vi "deleteWrite command description.vi"(8 "error in (no error)":errorcluster, 10 "command description":string, 11 "Help in":refnum<class "Help.lvclass">) -> (0 "error out":errorcluster, 3 "Help out":refnum<class "Help.lvclass">)   [LabVIEW 2019]
uses:
  Help.lvclass
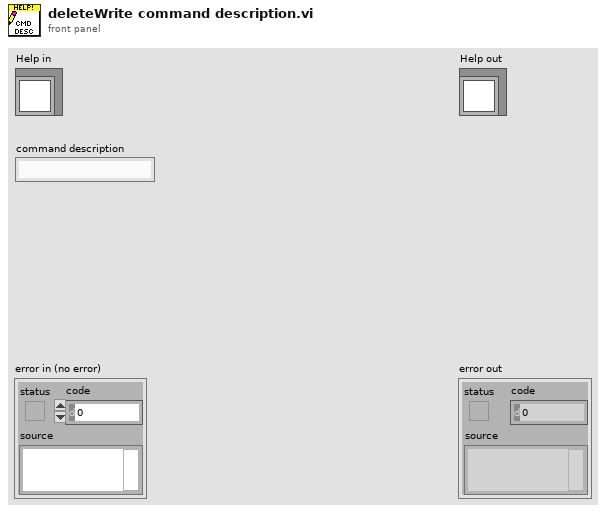
[diagram p1: front panel]
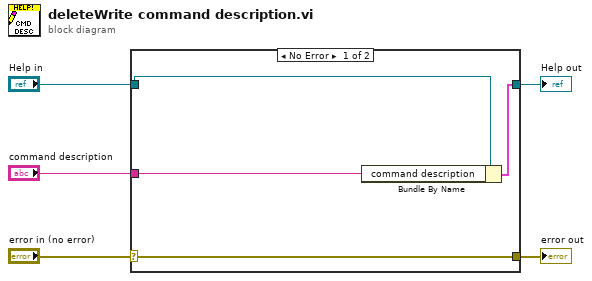
[diagram p0: block diagram]
diagram:
  n1 = case shown="No Error" "error in (no error)" {
    selector: "error in (no error)" -> [w9 w10]
    tunnel: [w9 w10] -> w4
    tunnel: [w7 w11] -> w2
    tunnel: "Help in" -> [w8 w11]
    tunnel: "command description" -> [w6 _]
    frame No Error {
      n2 = Bundle By Name(cluster=w8, "command description"=w6) -> (w7:cluster{})
    }
    frame Error {
    }
  }
  "error out" <- w4
  "Help out" <- w2
